vi "Create.vi"(8 "error in":errorcluster, 10 "reset":bool, 11 "option string":string) -> (0 "error out":errorcluster, 3 "session factory out":refnum<class "Session Factory.lvclass">)   [LabVIEW 2020, in "NI Session Management niScope.lvlib" / "Session Factory.lvclass"]
uses:
  Session Factory.lvclass
  Session Factory.lvclass/Session Factory.ctl
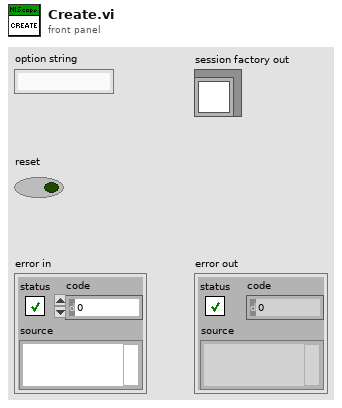
[diagram p1: front panel]
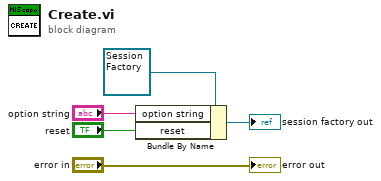
[diagram p0: block diagram]
diagram:
  n1 = Bundle By Name(cluster=refnum<class "Session Factory.lvclass"> refnum ("Instrument in"), "option string"="option string", "reset"="reset") -> (→"session factory out":refnum<class "Session Factory.lvclass">)
  "error out" <- "error in"
